vi "8 or 16 tubes.vi"() -> ()   [LabVIEW 2020]
panel:
  in  "8 tubes":bool
  out "CURRENT STATUS:\nThere are 16 tubes [RED]\nThere are 8 tubes [GREEN]":bool
  # "DO NOT SAVE ANYTHING WHEN CLOSING PROGRAM"
  # "^^ INITIALIZE HERE ^^"
  # "16 tubes"
  # "Flip down  for 8 tubes, up for 16\nPress white arrow in top left to initialize"
  # "8 tubes"
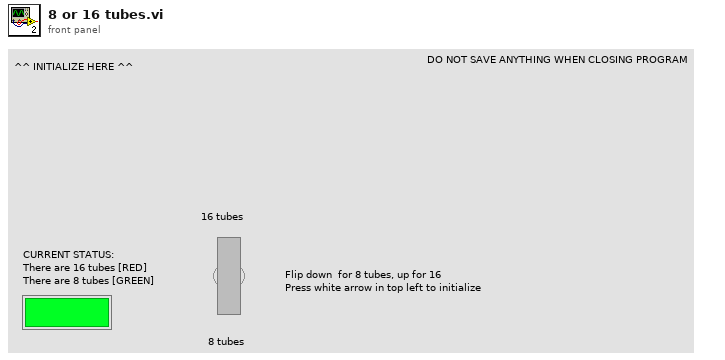
[diagram p1: front panel]
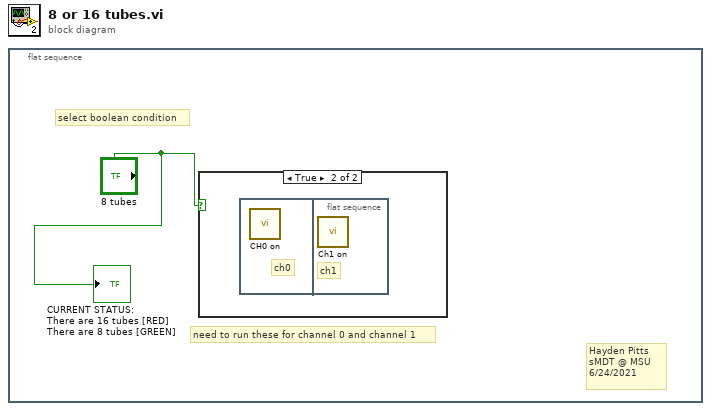
[diagram p0: block diagram]
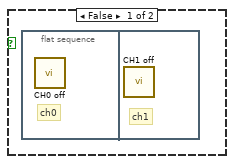
[diagram p2: hidden frame]
diagram:
  n1 = flat-sequence {
    frame #0 {
      # "Hayden Pitts\nsMDT @ MSU \n6/24/2021"
      # "select boolean condition"
      # "need to run these for channel 0 and channel 1"
      n2 = case shown="True" "8 tubes" {
        frame False {
          n3 = flat-sequence {
            frame #0 {
              # "ch0"
              n4 = call "CH0 off.vi"() -> ()  [unwired: 2 in, 1 out]
            }
            frame #1 {
              # "ch1"
              n5 = call "CH1 off.vi"() -> ()  [unwired: 2 in, 1 out]
            }
          }
        }
        frame True {
          n6 = flat-sequence {
            frame #0 {
              # "ch0"
              n7 = call "CH0 on.vi"() -> ()  [unwired: 2 in, 1 out]
            }
            frame #1 {
              # "ch1"
              n8 = call "Ch1 on.vi"() -> ()  [unwired: 2 in, 1 out]
            }
          }
        }
      }
      "CURRENT STATUS:\nThere are 16 tubes [RED]\nThere are 8 tubes [GREEN]" <- "8 tubes"
    }
  }
